vi "CRD CVT.vi"(8 "error in":errorcluster, 11 "Controller in":refnum<class "Controller.lvclass">) -> (0 "error out":errorcluster, 3 "Controller out":refnum<class "Controller.lvclass">)   [LabVIEW 2014, in "Controller.lvlib" / "Controller.lvclass"]
uses:
  Controller.lvclass
  <vilib>/Utility/config.llb/Config Data RefNum.ctl
  <vilib>/Utility/config.llb/Read Key (String).vi
  <vilib>/Utility/config.llb/Read Key (Double).vi
  <vilib>/Utility/config.llb/NI_LVConfig.lvlib
panel:
  in  "CfgRef":T1
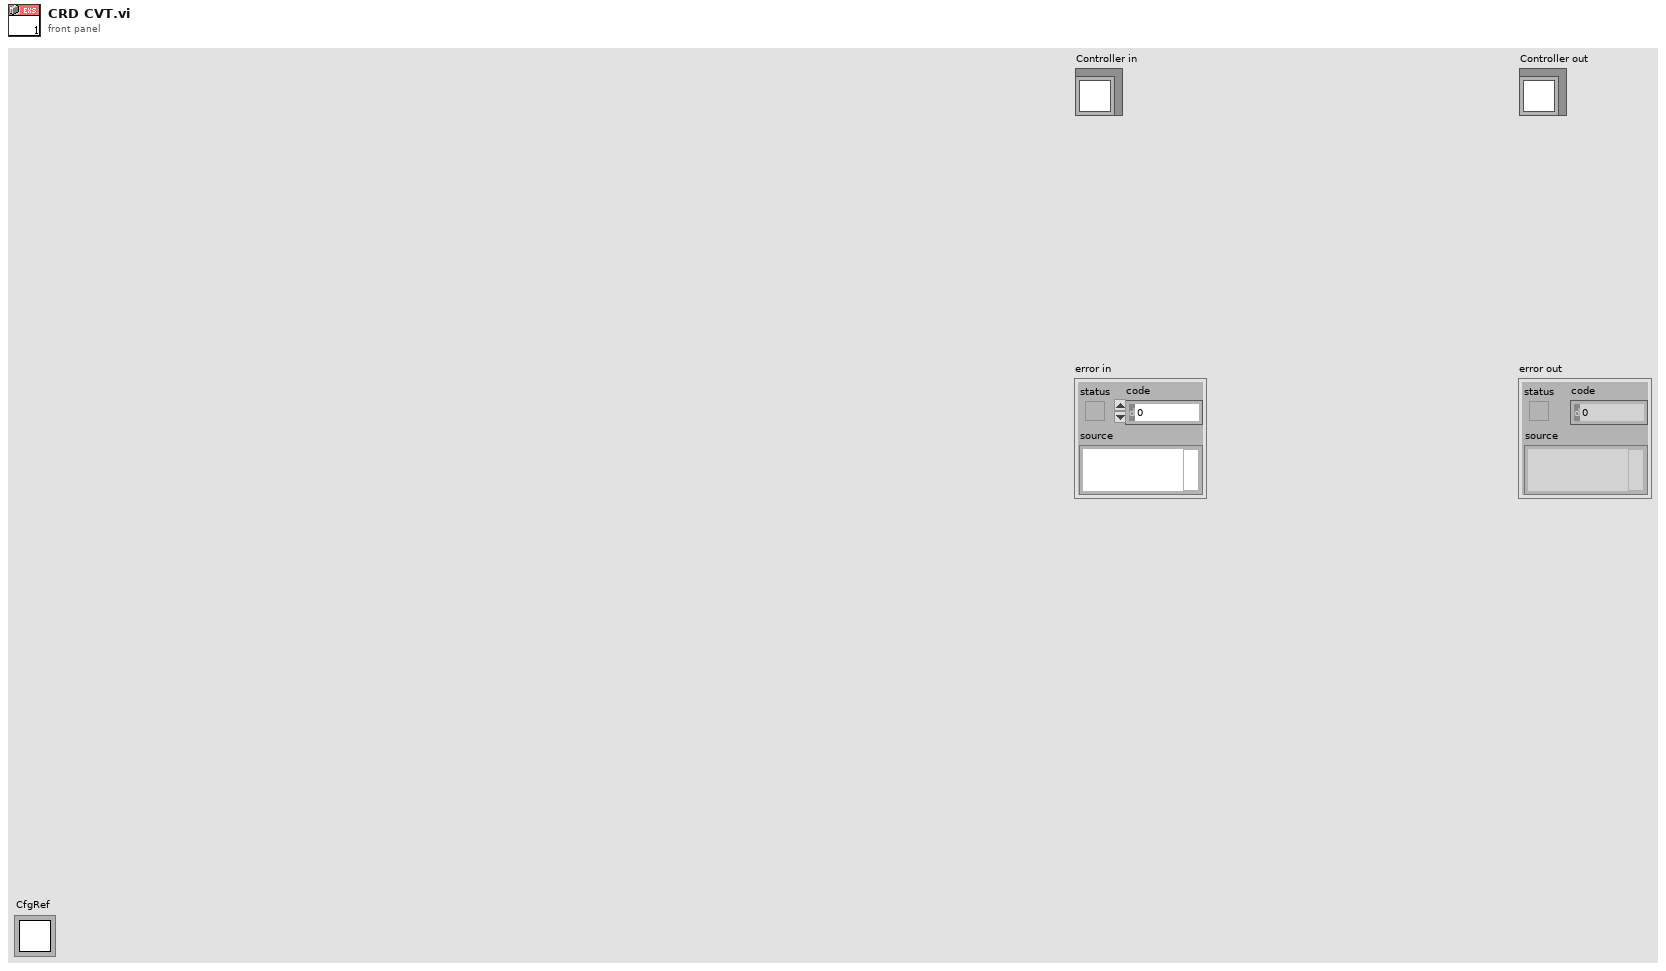
[diagram p1: front panel]
types:
  T1 = typedef "NI_LVConfig.lvlib/Config Data RefNum.ctl" = refnum<k1>
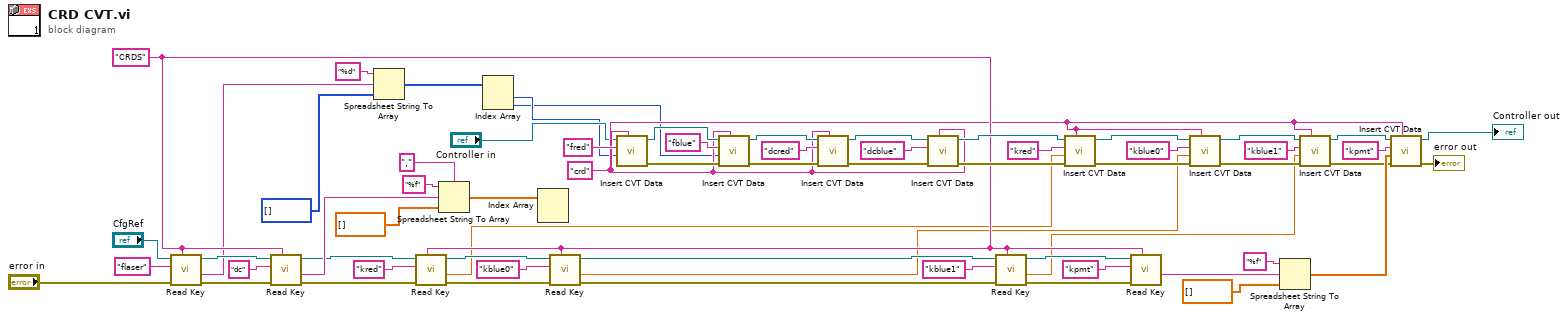
[diagram p0: block diagram]
diagram:
  w23 = "crd" ("Group")
  w29 = "CRDS" ("section")
  n1 = call-poly <vilib>:"Read Key.vi"("section"=w29, "error in (no error)"="error in", "key"="flaser", "refnum"="CfgRef") -> ("error out"=w50:errorcluster, "value"=w6:string, "refnum out"=w51:T1)  [unwired: 4 in, 1 out]
  n2 = call-poly <vilib>:"Read Key.vi"("section"=w29, "error in (no error)"=w50, "key"="dc", "refnum"=w51) -> ("error out"=w43:errorcluster, "value"=w45:string, "refnum out"=w44:T1)  [unwired: 4 in, 1 out]
  n3 = Spreadsheet String To Array(format string="%d", spreadsheet string=w6, array type (2D Dbl)=i16[] []) -> (array=w7:i16[])  [unwired: 1 in]
  n4 = call-poly <vilib>:"Read Key.vi"("section"=w29, "error in (no error)"=w43, "key"="kred" ("section"), "refnum"=w44) -> ("error out"=w32:errorcluster, "value"=w3:dbl, "refnum out"=w33:T1)  [unwired: 4 in, 1 out]
  n5 = Spreadsheet String To Array(delimiter (Tab)=",", format string="%f", spreadsheet string=w45, array type (2D Dbl)=sgl[] []) -> (array=w34:sgl[])
  n6 = Index Array(array=w7) -> (element #1=w5:i16, element #2=w4:i16)  [unwired: 2 in]
  n7 = Index Array(array=w34) -> ()  [unwired: 2 in, 2 out]
  n8 = call-poly <vilib>:"Read Key.vi"("section"=w29, "error in (no error)"=w32, "key"="kblue0", "refnum"=w33) -> ("error out"=w30:errorcluster, "value"=w15:dbl, "refnum out"=w31:T1)  [unwired: 4 in, 1 out]
  n9 = call "Insert CVT Data.vi"("Group"=w23, "Data"=w5, "tag"="fred" ("Tag Name"), "Controller in"="Controller in") -> ("error out"=w54:errorcluster, "Controller out"=w58:refnum<class "Controller.lvclass">)  [unwired: 6 in]
  n10 = call "Insert CVT Data.vi"("Group"=w23, "error in"=w54, "Data"=w4, "tag"="fblue" ("Tag Name"), "Controller in"=w58) -> ("error out"=w38:errorcluster, "Controller out"=w42:refnum<class "Controller.lvclass">)  [unwired: 5 in]
  n11 = call "Insert CVT Data.vi"("Group"=w23, "error in"=w38, "tag"="dcred", "Controller in"=w42) -> ("error out"=w39:errorcluster, "Controller out"=w41:refnum<class "Controller.lvclass">)  [unwired: 6 in]
  n12 = call "Insert CVT Data.vi"("Group"=w23, "error in"=w39, "tag"="dcblue", "Controller in"=w41) -> ("error out"=w37:errorcluster, "Controller out"=w40:refnum<class "Controller.lvclass">)  [unwired: 6 in]
  n13 = call-poly <vilib>:"Read Key.vi"("section"=w29, "error in (no error)"=w30, "key"="kblue1", "refnum"=w31) -> ("error out"=w27:errorcluster, "value"=w14:dbl, "refnum out"=w28:T1)  [unwired: 4 in, 1 out]
  n14 = call "Insert CVT Data.vi"("Group"=w23, "error in"=w37, "Data"=w3, "tag"="kred" ("Tag Name"), "Controller in"=w40) -> ("error out"=w20:errorcluster, "Controller out"=w24:refnum<class "Controller.lvclass">)  [unwired: 5 in]
  n15 = call-poly <vilib>:"Read Key.vi"("section"=w29, "error in (no error)"=w27, "key"="kpmt" ("section"), "refnum"=w28) -> ("value"=w11:string)  [unwired: 4 in, 3 out]
  n16 = call "Insert CVT Data.vi"("Group"=w23, "error in"=w20, "Data"=w15, "tag"="kblue0", "Controller in"=w24) -> ("error out"=w19:errorcluster, "Controller out"=w22:refnum<class "Controller.lvclass">)  [unwired: 5 in]
  n17 = Spreadsheet String To Array(format string="%f", spreadsheet string=w11, array type (2D Dbl)=sgl[] []) -> (array=w55:sgl[])  [unwired: 1 in]
  n18 = call "Insert CVT Data.vi"("Group"=w23, "error in"=w19, "Data"=w14, "tag"="kblue1", "Controller in"=w22) -> ("error out"=w18:errorcluster, "Controller out"=w21:refnum<class "Controller.lvclass">)  [unwired: 5 in]
  n19 = call "Insert CVT Data.vi"("Group"=w23, "error in"=w18, "Data"=w55, "tag"="kpmt" ("Tag Name"), "Controller in"=w21) -> ("error out"=→"error out":errorcluster, "Controller out"=→"Controller out":refnum<class "Controller.lvclass">)  [unwired: 5 in]
